vi "DB Tools Move To Record N.vi"   [LabVIEW 2012, in "NI_Database_API_64.lvlib"]
doc: "Moves the cursor to point to record <B>n</B> in the recordset. To move the cursor to the last record, set <B>n</B> to -1. You cannot use this VI with a forward-only cursor. Wire data to the reference input to determine the polymorphic instance to use or manually select the instance."
uses:
  NI_Database_API_64.lvlib
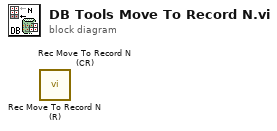
[diagram p0: block diagram]
diagram:
  n1 = call "Rec Move To Record N (R).vi"() -> ()  [unwired: 10 in, 2 out]
  n2 = call "Rec Move To Record N (CR).vi"() -> ()  [unwired: 10 in, 2 out]
